vi "TimeInterpRotation_AddSample.vi"(9 "RotationValue":T1={"VALUE"=0.0, "COS"=1.0, "SIN"=0.0} {"SIN" format="%13.4f"; "COS" format="%13.4f"; "VALUE" format="%13.4f"}, 10 "TimeStamp":dbl, 11 "in TimeInterpRotation":T2 {"RotationValues"."SIN" format="%13.4f"; "RotationValues"."COS" format="%13.4f"; "RotationValues"."VALUE" format="%13.4f"}) -> (0 "Error":bool, 3 "out TimeInterpRotation":T2 {"RotationValues"."SIN" format="%13.4f"; "RotationValues"."COS" format="%13.4f"; "RotationValues"."VALUE" format="%13.4f"})   [LabVIEW 2019, in "Trajectory_Library.lvlib"]
doc: "Insert new X, Y pair into an existing Function Generator data cluster.\n\nInputs:\n - \n\nOutputs:\n - Function Generator -- Created data structure"
uses:
  ROTATION2D.ctl
  Trajectory_Library.lvlib
  <vilib>/gmath/NI_Gmath.lvlib
  TIME_INTERPOLATABLE_ROTATION.ctl
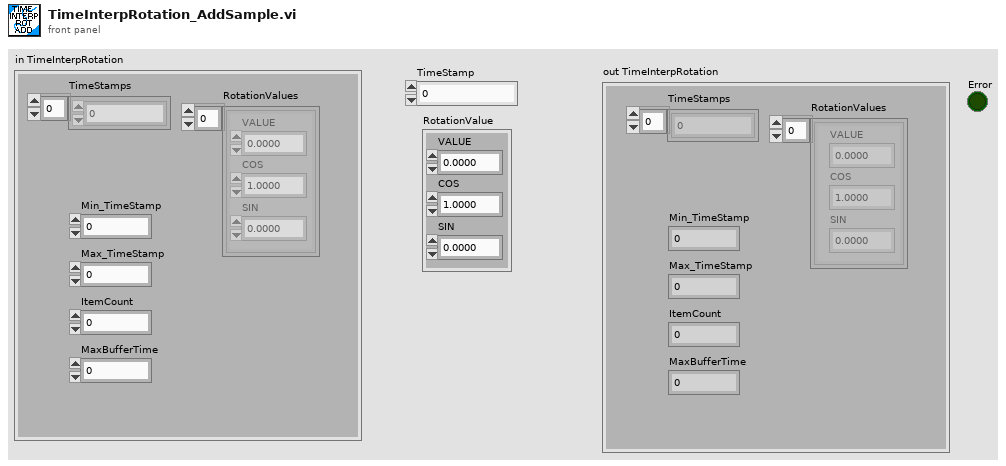
[diagram p1: front panel]
types:
  T1 = typedef "Trajectory_Library.lvlib/ROTATION2D.ctl" = cluster{"VALUE":dbl, "COS":dbl, "SIN":dbl}
  T2 = typedef "Trajectory_Library.lvlib/TIME_INTERPOLATABLE_ROTATION.ctl" = cluster{"TimeStamps":dbl[], "RotationValues":T1[], "Min_TimeStamp":dbl, "Max_TimeStamp":dbl, "ItemCount":i32, "MaxBufferTime":dbl}
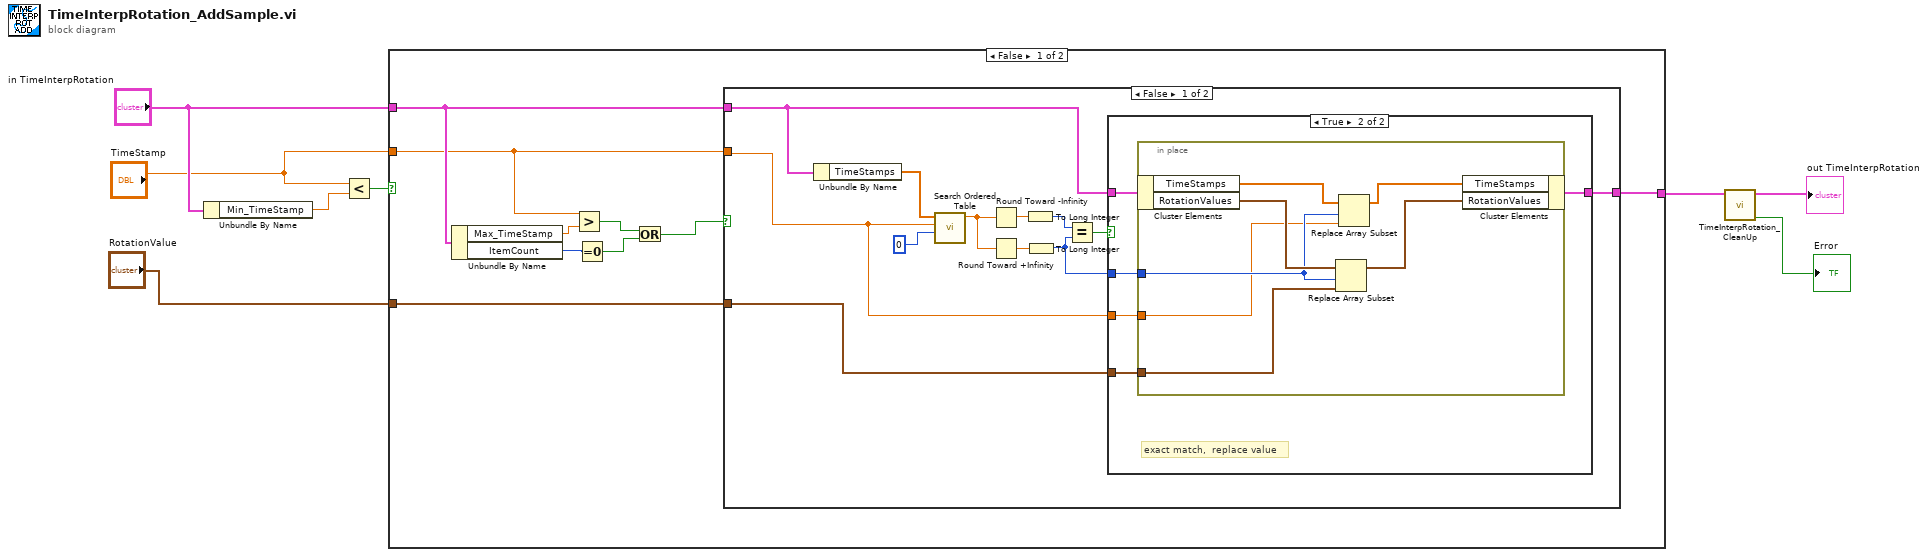
[diagram p0: block diagram]
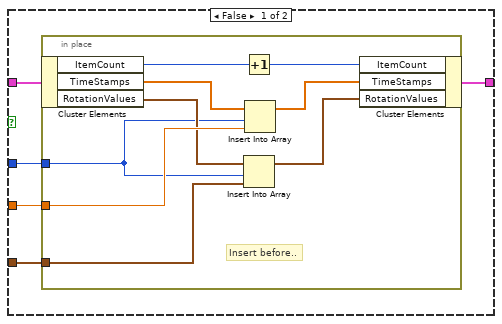
[diagram p2: hidden frame]
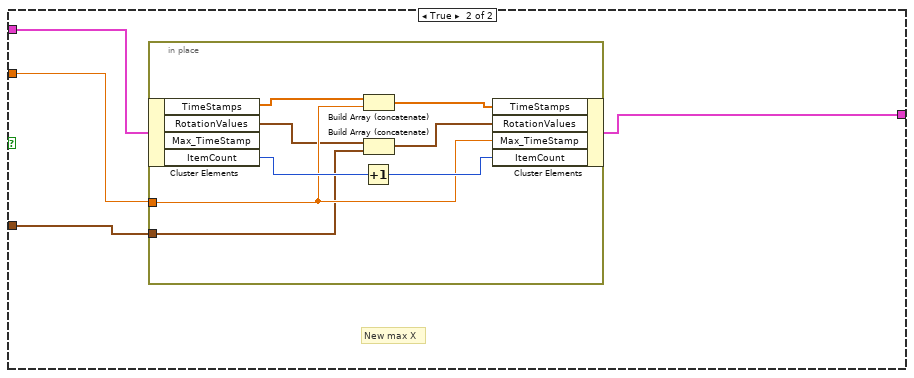
[diagram p3: hidden frame]
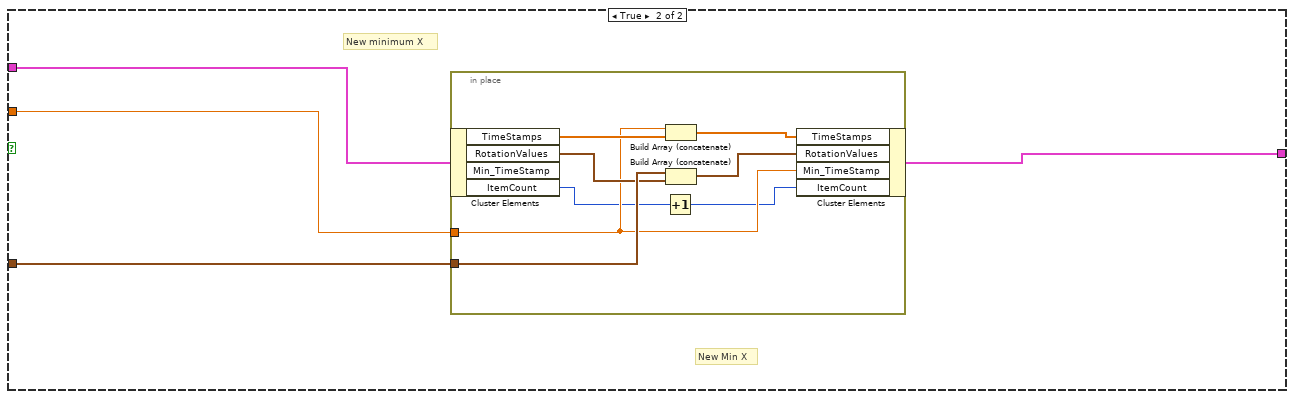
[diagram p4: hidden frame]
diagram:
  n1 = Unbundle By Name("in TimeInterpRotation") -> ("Min_TimeStamp"=w8:dbl)
  n2 = Less?(x="TimeStamp", y=w8) -> (x < y?=w7:bool)
  n3 = case shown="False" w7 {
    tunnel: "in TimeInterpRotation" -> [w16 w71]
    tunnel: "TimeStamp" -> [w14 w70]
    tunnel: "RotationValue" -> [w13 w69]
    tunnel: [w15 w68] -> w3
    frame False {
      n4 = Unbundle By Name(w16) -> ("Max_TimeStamp"=w17:dbl, "ItemCount"=w12:i32)
      n5 = Greater?(x=w14, y=w17) -> (0:w11:bool)
      n6 = Equal To 0?(x=w12) -> (x = 0?=w10:bool)
      n7 = Or(x=w11, y=w10) -> (x .or. y?=w9:bool)
      n8 = case shown="False" w9 {
        tunnel: w16 -> [w22 w59]
        tunnel: [w18 w58] -> w15
        tunnel: w14 -> [w20 w57]
        tunnel: w13 -> [w19 w56]
        frame False {
          n9 = Unbundle By Name(w22) -> ("TimeStamps"=w28:dbl[])
          n10 = call <vilib>:"Search Ordered Table.vi"("starting index"=0, "x value"=w20, "ordered x array"=w28) -> ("fractional index"=w27:dbl)  [unwired: 8 in]
          n11 = Round Toward -Infinity(1:w27) -> (0:w25:dbl)
          n12 = Round Toward +Infinity(x=w27) -> (ceil(x): smallest int >= x=w26:dbl)
          n13 = To Long Integer(number=w25) -> (32bit integer=w24:i32)
          n14 = To Long Integer(number=w26) -> (32bit integer=w21:i32)
          n15 = Equal?(x=w24, y=w21) -> (x = y?=w23:bool)
          n16 = case shown="True" w23 {
            tunnel: w22 -> [w31 w48]
            tunnel: w21 -> [w34 w47]
            tunnel: w20 -> [w33 w46]
            tunnel: w19 -> [w32 w45]
            tunnel: [w30 w44] -> w18
            frame False {
              n17 = in-place {
                in-place-border: w34 -> [w38]
                in-place-border: w33 -> [w40]
                in-place-border: w32 -> [w37]
                # "Insert before.."
                n18 = in-place-cluster #1(w31) -> ("ItemCount"=w43:i32, "TimeStamps"=w41:dbl[], "RotationValues"=w39:T1[])
                n19 = Increment(x=w43) -> (x+1=w42:i32)
                n20 = Insert Into Array(array=w39, index=w38, new element=w37) -> (w35:T1[])
                n21 = Insert Into Array(array=w41, index=w38, new element=w40) -> (w36:dbl[])
                n22 = in-place-cluster #1("ItemCount"=w42, "TimeStamps"=w36, "RotationValues"=w35) -> (w30:T2)
              }
            }
            frame True {
              # "exact match,  replace value"
              n23 = in-place {
                in-place-border: w47 -> [w53]
                in-place-border: w46 -> [w52]
                in-place-border: w45 -> [w51]
                n24 = in-place-cluster #2(w48) -> ("TimeStamps"=w55:dbl[], "RotationValues"=w54:T1[])
                n25 = Replace Array Subset(array=w54, new element=w51, index=w53) -> (w49:T1[])
                n26 = Replace Array Subset(array=w55, new element=w52, index=w53) -> (w50:dbl[])
                n27 = in-place-cluster #2("TimeStamps"=w50, "RotationValues"=w49) -> (w44:T2)
              }
            }
          }
        }
        frame True {
          # "New max X"
          n28 = in-place {
            in-place-border: w57 -> [w63]
            in-place-border: w56 -> [w60]
            n29 = in-place-cluster #3(w59) -> ("TimeStamps"=w62:dbl[], "RotationValues"=w61:T1[], "ItemCount"=w65:i32)  [unwired: 1 out]
            n30 = Increment(x=w65) -> (x+1=w64:i32)
            n31 = Build Array (concatenate)(w62, w63) -> (w67:dbl[])
            n32 = Build Array (concatenate)(w61, w60) -> (w66:T1[])
            n33 = in-place-cluster #3("TimeStamps"=w67, "RotationValues"=w66, "Max_TimeStamp"=w63, "ItemCount"=w64) -> (w58:T2)
          }
        }
      }
    }
    frame True {
      # "New Min X"
      # "New minimum X"
      n34 = in-place {
        in-place-border: w70 -> [w74]
        in-place-border: w69 -> [w79]
        n35 = in-place-cluster #4(w71) -> ("TimeStamps"=w78:dbl[], "RotationValues"=w75:T1[], "ItemCount"=w73:i32)  [unwired: 1 out]
        n36 = Increment(x=w73) -> (x+1=w72:i32)
        n37 = Build Array (concatenate)(w74, w78) -> (w77:dbl[])
        n38 = Build Array (concatenate)(w79, w75) -> (w76:T1[])
        n39 = in-place-cluster #4("TimeStamps"=w77, "RotationValues"=w76, "Min_TimeStamp"=w74, "ItemCount"=w72) -> (w68:T2)
      }
    }
  }
  n40 = call "TimeInterpRotation_CleanUp.vi"("in TimeInterpRotation"=w3) -> ("Error"=→"Error":bool, "out TimeInterpRotation"=→"out TimeInterpRotation":T2)  [unwired: 9 in]
